vi "20200106_Digital - Continuous Output.vi"() -> ()   [LabVIEW 2021]
doc: "This example demonstrates how to continuously re-generate digital output data. That output is hardware timed, so each sample is output on the next tick of the sample clock.\n\nSome hardware (e.g. M Series DAQ) must use an external sample clock for digital tasks. To view a complete list of available sample clock sources, consult the Device Routes table in Measurement and Automation Explorer.\n\nFor instructions on how to connect your signals to the DAQ device, refer to your device documentation."
uses:
  <vilib>/Utility/error.llb/DialogType.ctl
  <vilib>/DAQmx/write.llb/DAQmx Write (Digital 1D U8 1Chan NSamp).vi
  <vilib>/DAQmx/create/channels.llb/DAQmx Create Channel (DO-Digital Output).vi
  <vilib>/DAQmx/configure/timing.llb/DAQmx Timing (Sample Clock).vi
  <vilib>/DAQmx/configure/trigger.llb/DAQmx Start Trigger (Digital Edge).vi
  <vilib>/DAQmx/configure/trigger.llb/DAQmx Start Trigger (Time).vi
  <vilib>/Utility/file.llb/Read Delimited Spreadsheet (I64).vi
  <vilib>/DAQmx/miscellaneous.llb/DAQmx Fill In Error Info.vi
  <resource>/objmgr/daqmx.rc
panel:
  in  "Line(s)":tag="Dev1/port0/line0:7"
  in  "Stop":bool
  in  "Trigger Type":T1(tab)
  in  "Edge":i32(ring)=10280 items=["Rising"=10280, "Falling"=10171]
  in  "Digital Trigger Source":tag="PFI1"
  in  "When":timestamp
  in  "Select Time\nManually":bool
  in  "Number of Samples":i32=1000
  in  "Sample Rate":dbl=1000.0
  in  "Sample Clock Source":tag="PFI0"
  out "Actual Sample Rate":dbl=1000.0 format="%0.2f"
  # "Channel Settings"
  # "Data to Write"
  # "Timing and Buffer Settings"
  # "Trigger Settings"
  # "To configure and use a start trigger you must have the necessary tab selected above.  Not all hardware supports triggering--refer to your device documentation for more info."
  # "If time is not manually set, task will begin after 10 seconds"
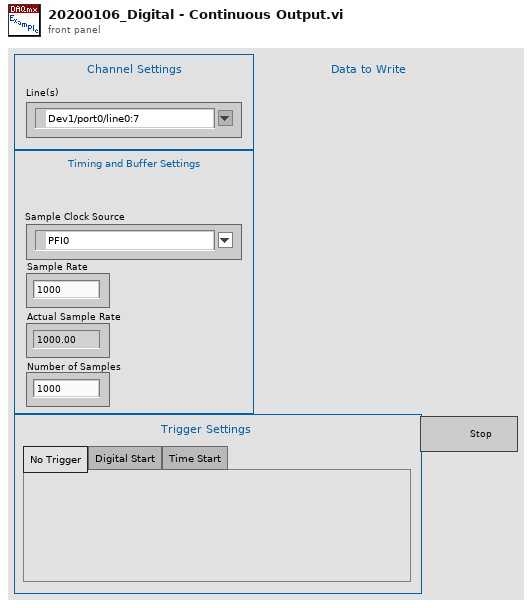
[diagram p1: front panel]
types:
  T1 = enum32{"No Trigger", "Digital Start", "Time Start"}
  T2 = typedef "DialogType.ctl" = u16
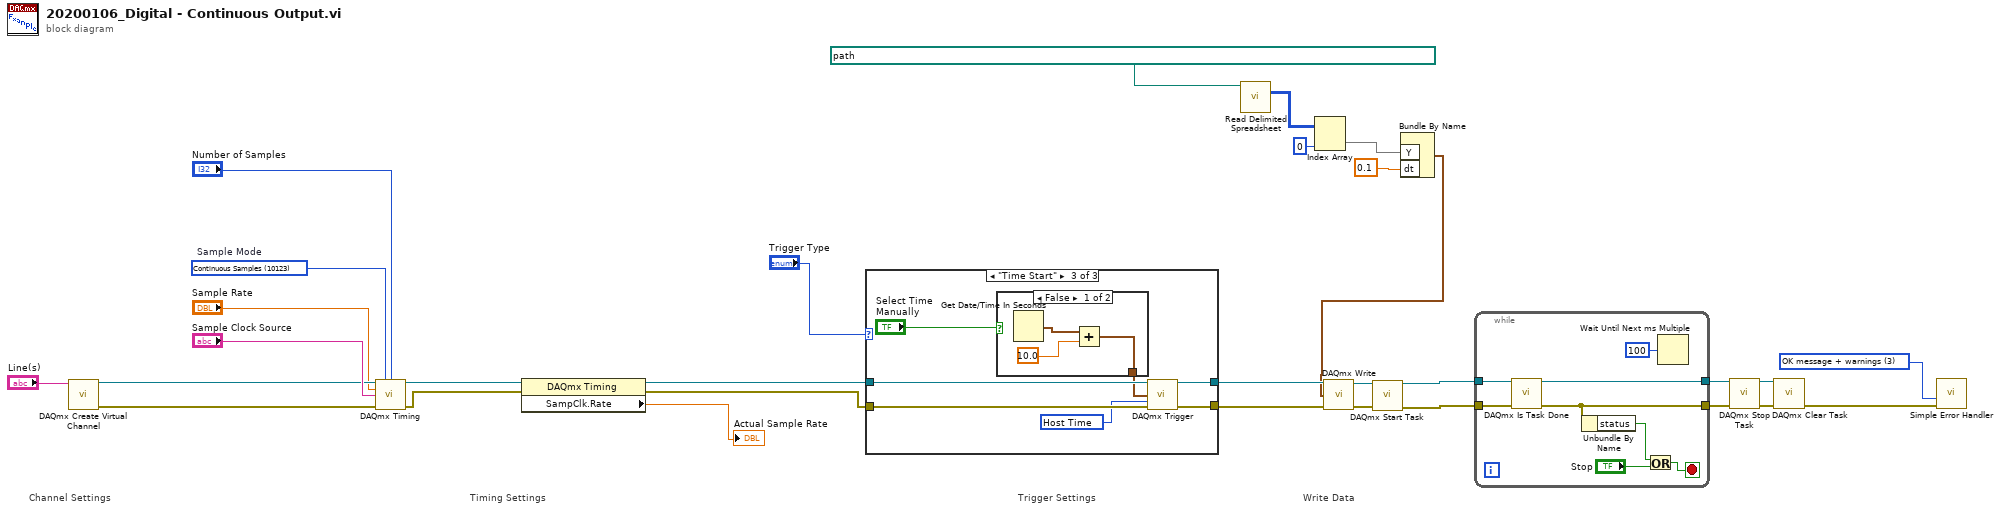
[diagram p0: block diagram]
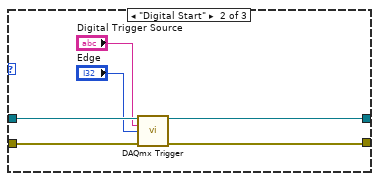
[diagram p3: hidden frame]
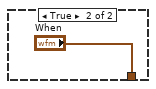
[diagram p4: hidden frame]
diagram:
  w7 = T2 3 items=["no dialog", "OK message", "continue or stop message", "OK message + warnings", "continue/stop + warnings"] ("type of dialog (OK msg:1)")
  w24 = 10123 items=["Finite Samples"=10178, "Continuous Samples"=10123, "Hardware Timed Single Point"=12522]  # Sample Mode
  # "Trigger Settings"
  # "Timing Settings"
  # "Write Data"
  # "Channel Settings"
  n1 = call-poly <vilib>:"DAQmx Create Virtual Channel.vi"("lines"="Line(s)") -> ("task out"=w28:refnum<k21>, "error out"=w27:errorcluster)  [unwired: 13 in]
  n2 = call-poly <vilib>:"DAQmx Timing.vi"("task/channels in"=w28, "sample mode"=w24, "samples per channel"="Number of Samples", "rate"="Sample Rate", "source"="Sample Clock Source", "error in"=w27) -> ("task out"=w23:refnum<k21>, "error out"=w22:errorcluster)  [unwired: 8 in]
  n3 = property class="DAQmx Timing"(reference=w23, error in=w22) -> (reference out=w20:refnum<k21>, error out=w19:errorcluster, "SampClk.Rate"=→"Actual Sample Rate":dbl)
  n4 = case shown="\"Time Start\"" "Trigger Type" {
    tunnel: w20 -> [w33 w39 w46]
    tunnel: w19 -> [w32 w38 w45]
    tunnel: [w33 w37 w44] -> w18
    tunnel: [w32 w36 w43] -> w17
    frame "No Trigger", Default {
    }
    frame "Digital Start" {
      n5 = call-poly <vilib>:"DAQmx Trigger.vi"("task/channels in"=w39, "source"="Digital Trigger Source", "edge"="Edge", "error in"=w38) -> ("task out"=w37:refnum<k21>, "error out"=w36:errorcluster)  [unwired: 10 in]
    }
    frame "Time Start" {
      w40 = 16126 items=["Host Time"=16126, "I/O Device Time"=16127] ("timescale")
      n6 = case shown="False" "Select Time\nManually" {
        tunnel: [w48 "When"] -> w41
        frame False {
          n7 = Get Date/Time In Seconds() -> (seconds since 1Jan1904=w49:timestamp)
          n8 = Add(x=w49, y=10.0) -> (x+y=w48:timestamp)
        }
        frame True {
        }
      }
      n9 = call-poly <vilib>:"DAQmx Trigger.vi"("task/channels in"=w46, "when"=w41, "timescale"=w40, "error in"=w45) -> ("task out"=w44:refnum<k21>, "error out"=w43:errorcluster)  [unwired: 10 in]
    }
  }
  n10 = call-poly <vilib>:"Read Delimited Spreadsheet.vi"("file path (dialog if empty)"=path "C:/Users/joe.kao/OneDrive - eCloudvalley Digital Technology/桌面/nPM1100_WaveformTable_Digital_LV.txt") -> ("all rows"=w5:i64[][])  [unwired: 9 in, 5 out]
  n11 = Index Array(array=w5, index (col)=0 ("disabled index (col)")) -> (element=w2:i64[])  [unwired: 1 in]
  n12 = Bundle By Name("Y"=w2, "dt"=0.1) -> (w1:waveform(i64))  [unwired: 1 in]
  n13 = call-poly <vilib>:"DAQmx Write.vi"("task/channels in"=w18, "data"=w1, "error in"=w17) -> ("task out"=w16:refnum<k21>, "error out"=w15:errorcluster)  [unwired: 10 in, 1 out]
  n14 = call <vilib>:"DAQmx Start Task.vi"("task/channels in"=w16, "error in"=w15) -> ("task out"=w14:refnum<k21>, "error out"=w13:errorcluster)  [unwired: 12 in]
  n15 = while {
    tunnel: w14 -> [w58]
    tunnel: w13 -> [w57]
    tunnel: [w54] -> w8
    tunnel: [w56] -> w9
    stop <- w51 stop-if-true
    n16 = call <vilib>:"DAQmx Is Task Done.vi"("task/channels in"=w58, "error in"=w57) -> ("task out"=w56:refnum<k21>, "error out"=w54:errorcluster)  [unwired: 11 in, 1 out]
    n17 = Unbundle By Name(w54) -> ("status"=w53:bool)
    n18 = Or(x=w53, y="Stop") -> (x .or. y?=w51:bool)
    n19 = Wait Until Next ms Multiple(millisecond multiple=u32 100) -> ()  [unwired: 1 out]
  }
  n20 = call <vilib>:"DAQmx Stop Task.vi"("task/channels in"=w9, "error in"=w8) -> ("task out"=w11:refnum<k21>, "error out"=w10:errorcluster)  [unwired: 12 in]
  n21 = call <vilib>:"DAQmx Clear Task.vi"("task in"=w11, "error in"=w10) -> ("error out"=w31:errorcluster)  [unwired: 13 in]
  n22 = call <vilib>:"Simple Error Handler.vi"("type of dialog (OK msg:1)"=w7, "error in (no error)"=w31) -> ()  [unwired: 3 in, 5 out]
